vi "Wait For Events in Idle-M.vi"(6 "Boiler Controls":T4 {"Fuel Control Valve Position (% Open)" scale=0.0..100.0 scale format="%#_5g"}, 7 "Boiler Status Indicators In":T1 {"Time Count" format="%.1f"}, 8 "error in (no error)":errorcluster, 9 "Boiler Simulation Controls":T2 {"Flame Sesnor Value (%)" scale=0.0..100.0}, 10 "Last State Before Idle":T3, 11 "Timer Ouput":T5) -> (0 "error out":errorcluster, 1 "Next State":T3, 2 "Cluster out":cluster{"Time Target (s)":dbl, "Reset":bool}, 3 "Boiler Status Indicators Out":T1 {"Time Count" format="%.1f"})   [LabVIEW 2020]
uses:
  Controls/Boiler States Enum-M.ctl
panel:
  # "Seconds"
  # "Seconds"
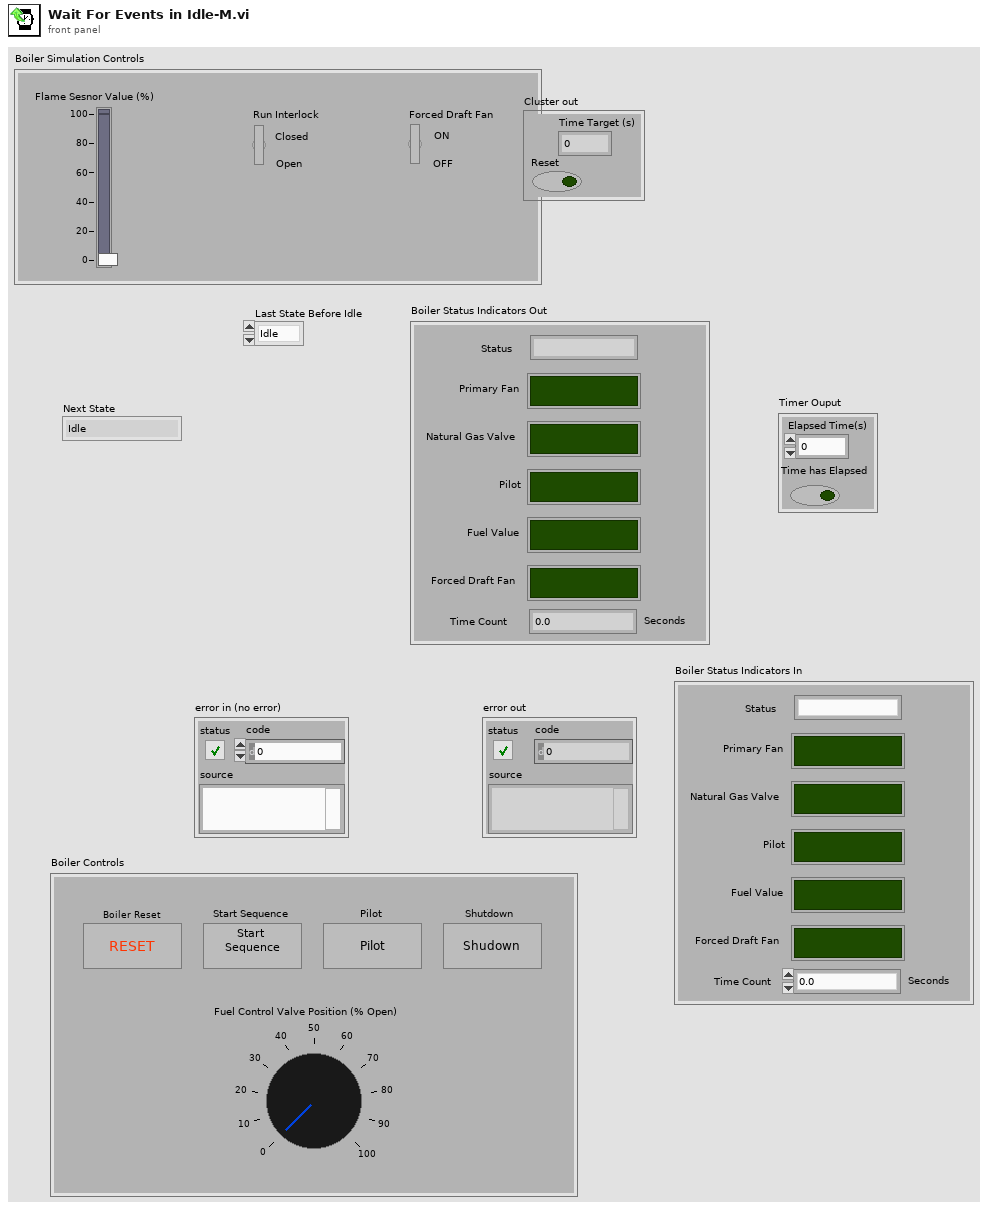
[diagram p1: front panel]
types:
  T1 = cluster{"Primary Fan":bool, "Natural Gas Valve":bool, "Pilot":bool, "Fuel Value":bool, "Forced Draft Fan":bool, "Time Count    ":dbl, "Status":string}
  T2 = cluster{"Flame Sesnor Value (%)":dbl, "Run Interlock":bool, "Forced Draft Fan":bool}
  T3 = typedef "Boiler States Enum-M.ctl" = enum16{"Idle", "Initialize", "Reset Lockout", "Pre-Purge", "Pre-Purge Complete", "Ignition", "Pilot", "Shutdown Purge Complete", "Shutdown Purge Start", "Run", "Pilot Proved", "Forced Draft Fan On"}
  T4 = cluster{"Shutdown":bool, "Pilot":bool, "Start Sequence":bool, "Fuel Control Valve Position (% Open)":dbl, "Boiler Reset":bool}
  T5 = cluster{"Time has Elapsed":bool, "Elapsed Time(s)":dbl}
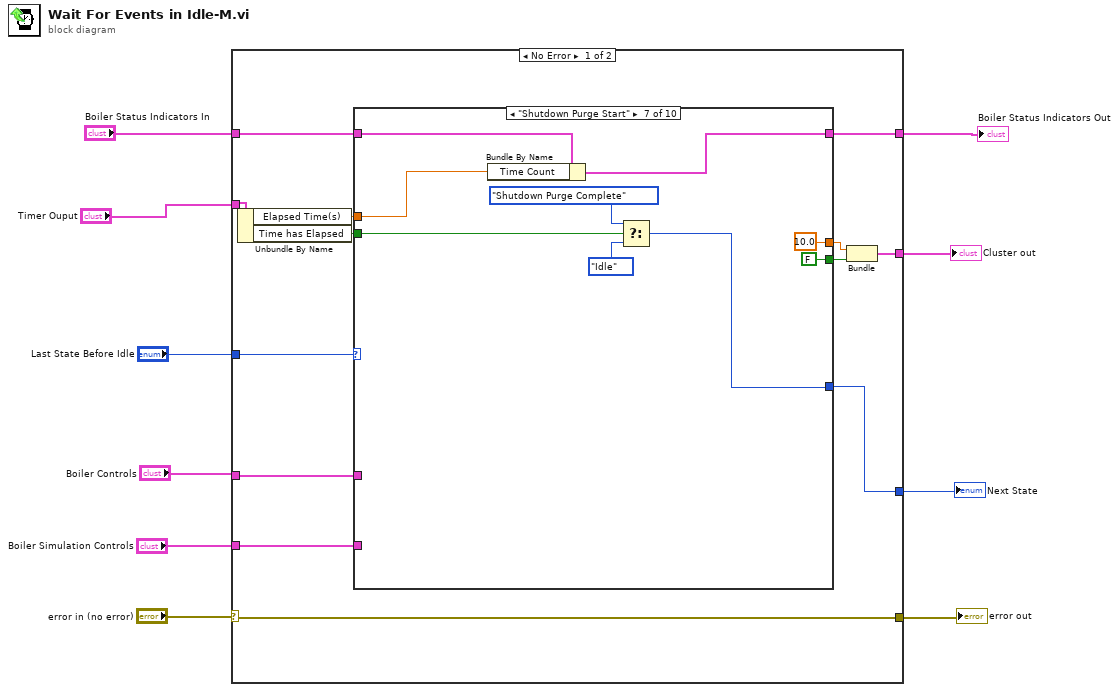
[diagram p0: block diagram]
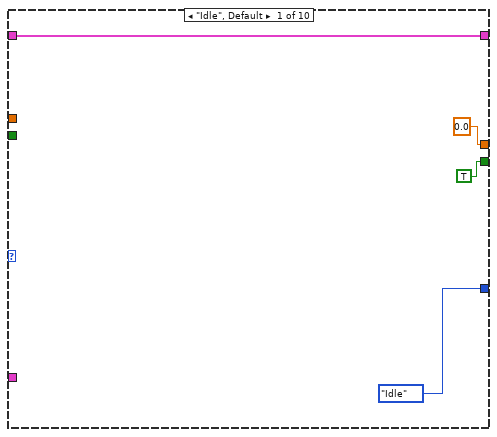
[diagram p2: hidden frame]
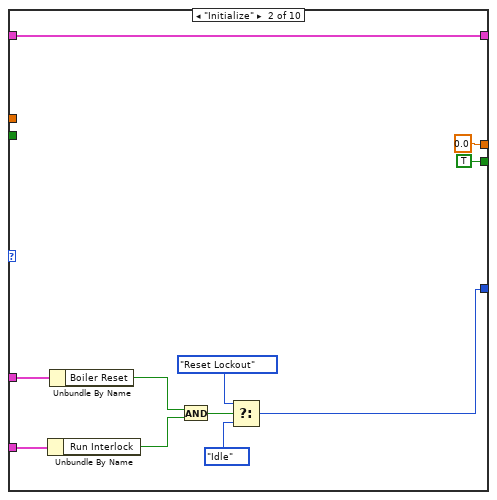
[diagram p3: hidden frame]
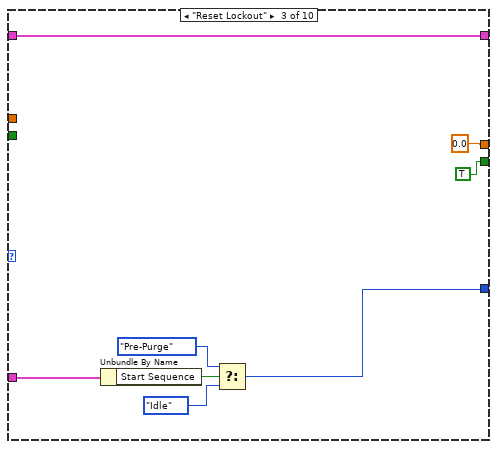
[diagram p4: hidden frame]
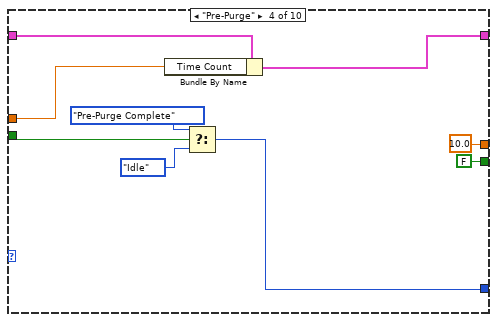
[diagram p5: hidden frame]
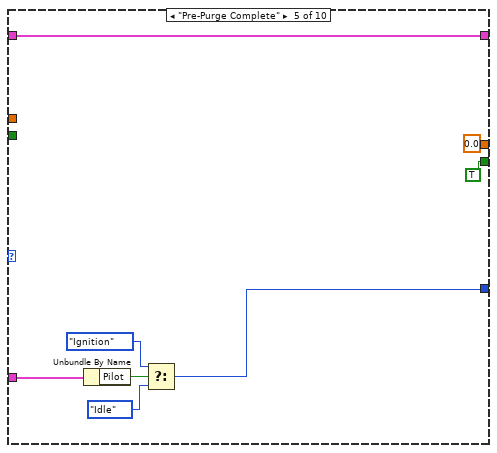
[diagram p6: hidden frame]
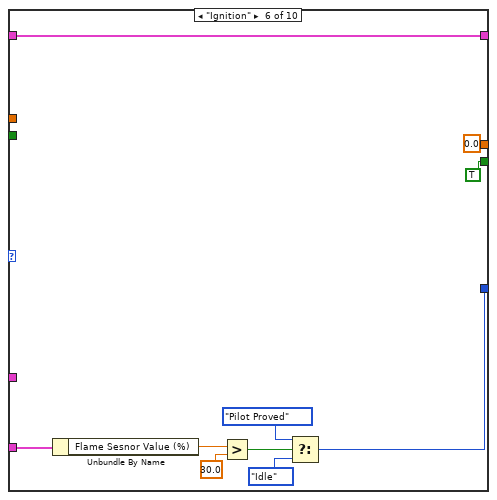
[diagram p7: hidden frame]
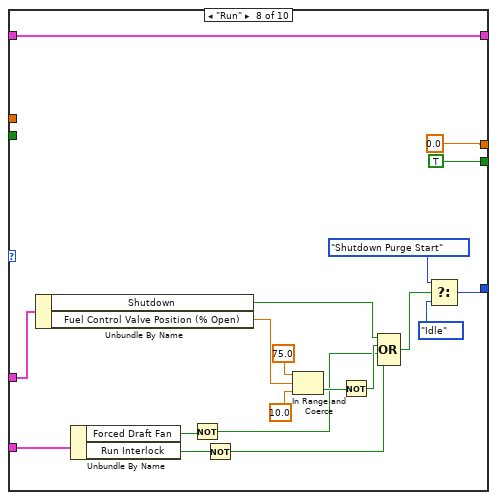
[diagram p8: hidden frame]
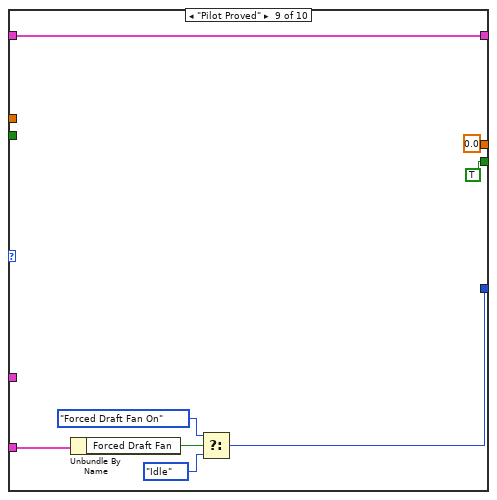
[diagram p9: hidden frame]
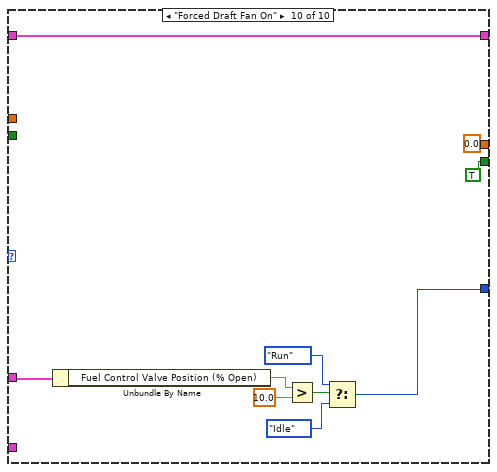
[diagram p10: hidden frame]
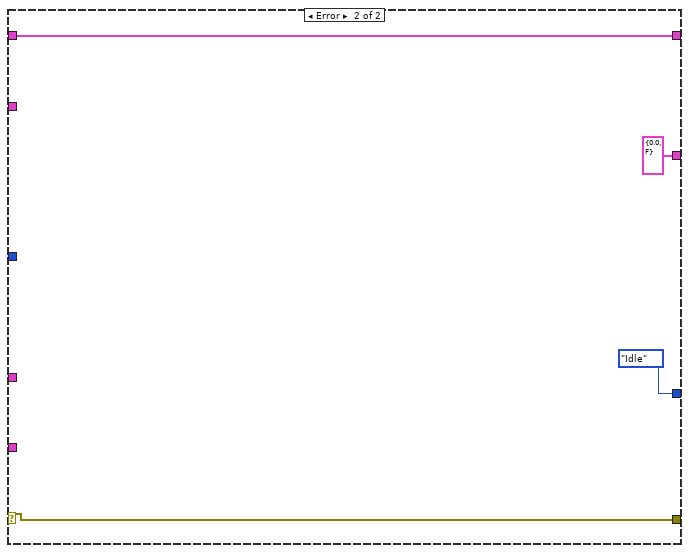
[diagram p11: hidden frame]
diagram:
  n1 = case shown="No Error" "error in (no error)" {
    selector: "error in (no error)" -> [w15 w123]
    tunnel: [w15 w123] -> w3
    tunnel: "Last State Before Idle" -> [w23 _]
    tunnel: "Boiler Status Indicators In" -> [w22 w122]
    tunnel: [w21 w122] -> w2
    tunnel: [w20 cluster{"Time Target (s)":dbl, "Reset":bool} {"Time Target (s)"=0.0, "Reset"=FALSE}] -> w5
    tunnel: "Boiler Controls" -> [w19 _]
    tunnel: [w18 Boiler_States_Enum-M."Idle" ("Last State Before Idle")] -> w7
    tunnel: "Boiler Simulation Controls" -> [w17 _]
    tunnel: "Timer Ouput" -> [w16 _]
    frame No Error {
      n2 = Unbundle By Name(w16) -> ("Elapsed Time(s)"=w14:dbl, "Time has Elapsed"=w13:bool)
      n3 = case shown="\"Shutdown Purge Start\"" w23 {
        tunnel: w22 -> [w25 w38 w39 w55 w56 w64 w82 w101 w109 w119]
        tunnel: [w25 w38 w39 w53 w56 w64 w81 w101 w109 w119] -> w21
        tunnel: [0.0 ("Time Target (s)") 0.0 ("Time Target (s)") 0.0 ("Time Target (s)") 10.0 ("Time Target (s)") 0.0 ("Time Target (s)") 0.0 ("Time Target (s)") 10.0 ("Time Target (s)") 0.0 ("Time Target (s)") 0.0 ("Time Target (s)") 0.0 ("Time Target (s)")] -> w11
        tunnel: [TRUE ("Reset") TRUE ("Reset") TRUE ("Reset") FALSE ("Reset") TRUE ("Reset") TRUE ("Reset") FALSE ("Reset") TRUE ("Reset") TRUE ("Reset") TRUE ("Reset")] -> w12
        tunnel: w19 -> [_ w35 w43 _ w63 _ _ w98 _ w118]
        tunnel: [Boiler_States_Enum-M."Idle" ("Last State Before Idle") w28 w40 w49 w59 w67 w76 w83 w106 w112] -> w18
        tunnel: w17 -> [_ w34 _ _ _ w73 _ w97 w108 _]
        tunnel: w14 -> [_ _ _ w54 _ _ w80 _ _ _]
        tunnel: w13 -> [_ _ _ w50 _ _ w79 _ _ _]
        frame "Idle", Default {
        }
        frame "Initialize" {
          n4 = Unbundle By Name(w34) -> ("Run Interlock"=w32:bool)
          n5 = Unbundle By Name(w35) -> ("Boiler Reset"=w33:bool)
          n6 = And(x=w33, y=w32) -> (x .and. y?=w31:bool)
          n7 = Select(t=Boiler_States_Enum-M."Reset Lockout" ("Last State Before Idle"), s=w31, f=Boiler_States_Enum-M."Idle" ("Last State Before Idle")) -> (s? t:f=w28:T3)
        }
        frame "Reset Lockout" {
          n8 = Unbundle By Name(w43) -> ("Start Sequence"=w46:bool)
          n9 = Select(t=Boiler_States_Enum-M."Pre-Purge" ("Last State Before Idle"), s=w46, f=Boiler_States_Enum-M."Idle" ("Last State Before Idle")) -> (s? t:f=w40:T3)
        }
        frame "Pre-Purge" {
          n10 = Bundle By Name(cluster=w55, "Time Count"=w54) -> (w53:T1)
          n11 = Select(t=Boiler_States_Enum-M."Pre-Purge Complete" ("Last State Before Idle"), s=w50, f=Boiler_States_Enum-M."Idle" ("Last State Before Idle")) -> (s? t:f=w49:T3)
        }
        frame "Pre-Purge Complete" {
          n12 = Unbundle By Name(w63) -> ("Pilot"=w62:bool)
          n13 = Select(t=Boiler_States_Enum-M."Ignition" ("Last State Before Idle"), s=w62, f=Boiler_States_Enum-M."Idle" ("Last State Before Idle")) -> (s? t:f=w59:T3)
        }
        frame "Ignition" {
          n14 = Unbundle By Name(w73) -> ("Flame Sesnor Value (%)"=w72:dbl)
          n15 = Greater?(x=w72, y=30.0) -> (0:w70:bool)
          n16 = Select(t=Boiler_States_Enum-M."Pilot Proved" ("Last State Before Idle"), s=w70, f=Boiler_States_Enum-M."Idle" ("Last State Before Idle")) -> (s? t:f=w67:T3)
        }
        frame "Shutdown Purge Start" {
          n17 = Bundle By Name(cluster=w82, "Time Count"=w80) -> (w81:T1)
          n18 = Select(t=Boiler_States_Enum-M."Shutdown Purge Complete" ("Last State Before Idle"), s=w79, f=Boiler_States_Enum-M."Idle" ("Last State Before Idle")) -> (s? t:f=w76:T3)
        }
        frame "Run" {
          n19 = Unbundle By Name(w98) -> ("Shutdown"=w90:bool, "Fuel Control Valve Position (% Open)"=w95:dbl)
          n20 = Unbundle By Name(w97) -> ("Forced Draft Fan"=w93:bool, "Run Interlock"=w91:bool)
          n21 = Not(x=w93) -> (.not. x?=w88:bool)
          n22 = Not(x=w91) -> (.not. x?=w87:bool)
          n23 = In Range and Coerce(upper limit=75.0, x=w95, lower limit=10.0) -> (In Range?=w92:bool)  [unwired: 1 out]
          n24 = Not(x=w92) -> (.not. x?=w89:bool)
          n25 = Compound Arithmetic op=OR(w90, w89, w88, w87) -> (w86:bool)
          n26 = Select(t=Boiler_States_Enum-M."Shutdown Purge Start" ("Last State Before Idle"), s=w86, f=Boiler_States_Enum-M."Idle" ("Last State Before Idle")) -> (s? t:f=w83:T3)
        }
        frame "Pilot Proved" {
          n27 = Unbundle By Name(w108) -> ("Forced Draft Fan"=w107:bool)
          n28 = Select(t=Boiler_States_Enum-M."Forced Draft Fan On" ("Last State Before Idle"), s=w107, f=Boiler_States_Enum-M."Idle" ("Last State Before Idle")) -> (s? t:f=w106:T3)
        }
        frame "Forced Draft Fan On" {
          n29 = Unbundle By Name(w118) -> ("Fuel Control Valve Position (% Open)"=w117:dbl)
          n30 = Greater?(x=w117, y=10.0) -> (0:w115:bool)
          n31 = Select(t=Boiler_States_Enum-M."Run" ("Last State Before Idle"), s=w115, f=Boiler_States_Enum-M."Idle" ("Last State Before Idle")) -> (s? t:f=w112:T3)
        }
      }
      n32 = Bundle("Time Target (s)"=w11, "Reset"=w12) -> (w20:cluster{"Time Target (s)":dbl, "Reset":bool})  [unwired: 1 in]
    }
    frame Error {
    }
  }
  "error out" <- w3
  "Next State" <- w7
  "Cluster out" <- w5
  "Boiler Status Indicators Out" <- w2
